vi "NI-SWITCH SwitchBlock Configuration.vi"(8 "error in (no error)":errorcluster, 11 "Reference In":refnum<k15>) -> (0 "error out":errorcluster, 1 "Analog Bus Array":string[](array[string]), 2 "Row Array":string[](array[string]), 3 "Reference out":refnum<k15>)   [LabVIEW 2019]
doc: "I. Description:\n\nThis is a subVI designed for use with NI SwitchBlock with NI-SWITCH. The purpose of this VI is to take in the NI SwitchBlock device, determine the number of rows and cards on the device, and generate a list of names for the rows and the analog bus lines on the NI SwitchBlock device\n\nII. Instructions for Running:\n\n1. Put your NI SWITCH reference into the control.\n2. Run the VI to produce two arrays of naming data for your NI SwitchBlock rows and analog buses.\n\nRefer to the NI Switches Help for the valid channel names and valid resource names for your switch module.\n\nIII. Block Diagram Steps:\n\n1.) Determine the model name, number of columns, and the number of rows from your NI SwitchBlock device.\n2.) Determine the number of cards on the NI SwitchBlock device by dividing the total number of columns, by the number of columns on each NI SwitchBlock card.\n3.) Use SwitchBlock Arrays.vi to find the names of the rows and analog buses on you device.\n\nIV. I/O Connections Overview:\n\nRefer to the NI Switches Getting Started Guide and NI Switches Help for information about connecting signals to your switch module."
uses:
  <resource>/objmgr/daqmx.rc
panel:
  out "Topology":string
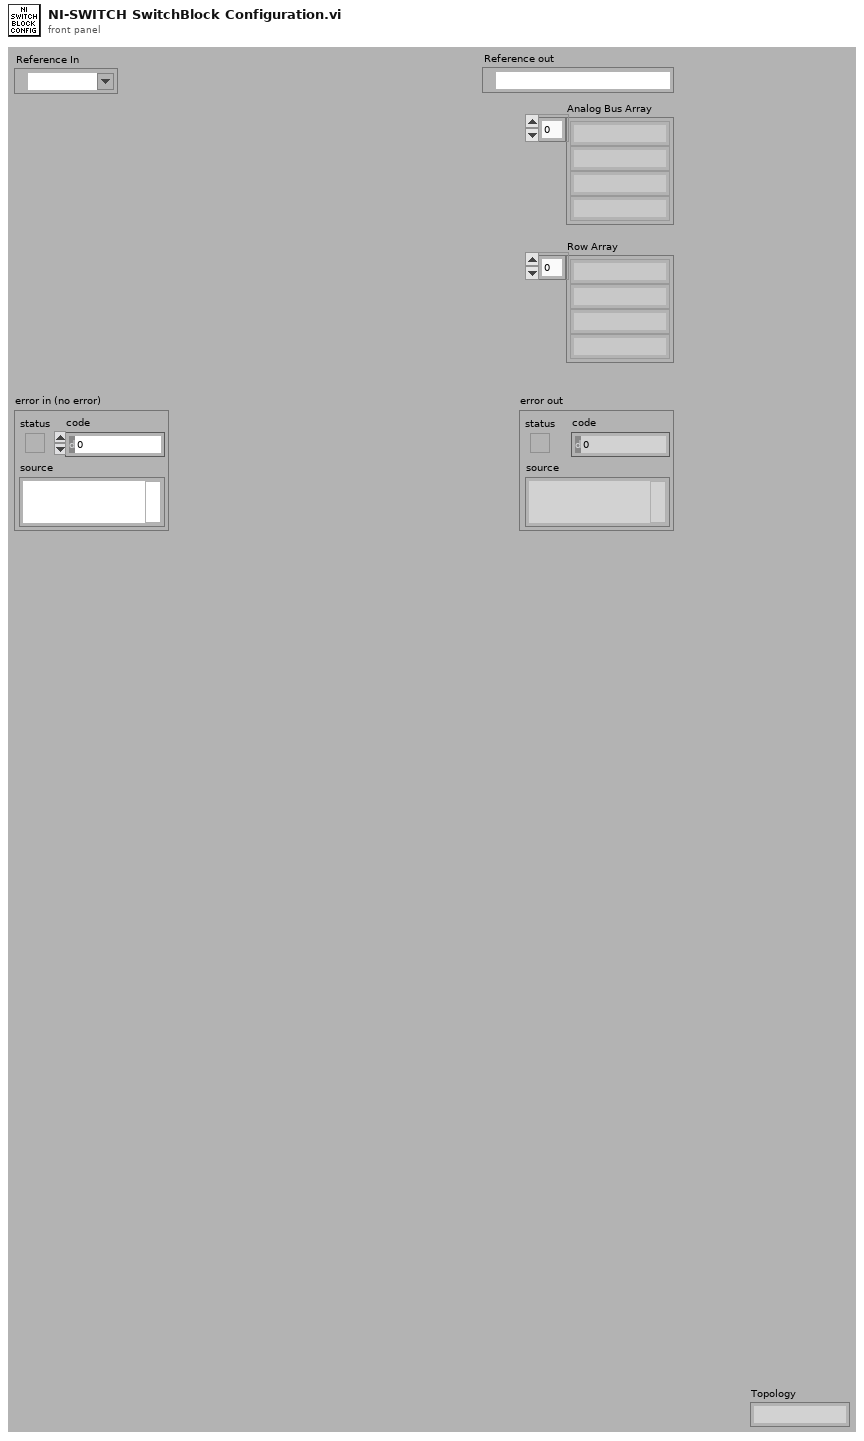
[diagram p1: front panel]
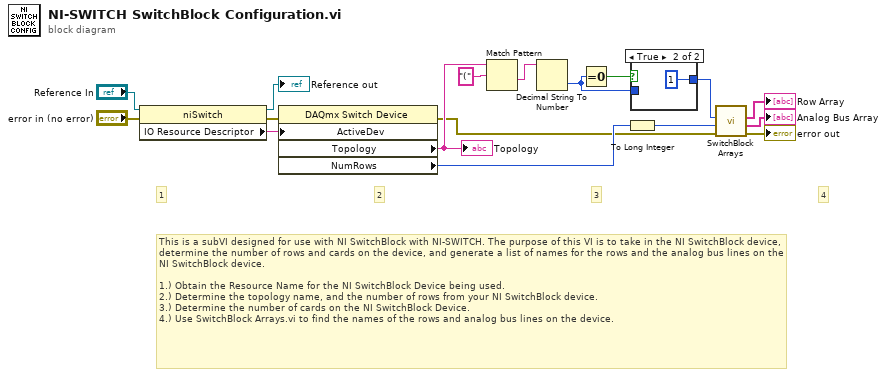
[diagram p0: block diagram]
diagram:
  # "4"
  # "3"
  # "2"
  # "1"
  # "This is a subVI designed for use with NI SwitchBlock with NI-SWITCH. The purpose of this VI is to take in the NI SwitchBlock device, determine the number of rows and cards on the device, and generate a list of names for the rows and the analog bus lines on the NI SwitchBlock device.\n\n1.) Obtain the Resource Name for the NI SwitchBlock Device being used.\n2.) Determine the topology name, and the number of rows from your NI SwitchBlock device.\n3.) Determine the number of cards on the NI SwitchBlock Device.\n4.) Use SwitchBlock Arrays.vi to find the names of the rows and analog bus lines on the device."
  n1 = property class="niSwitch"(reference="Reference In", error in="error in (no error)") -> (reference out=→"Reference out":refnum<k15>, error out=w4:errorcluster, "IO Resource Descriptor"=w5:string)
  n2 = property class="DAQmx Switch Device"(error in=w4, "ActiveDev"=w5) -> (error out=w1:errorcluster, "Topology"=w7:string, "NumRows"=w6:u32)  [unwired: 1 in, 1 out]
  "Topology" <- w7
  n3 = Match Pattern(string=w7, regular expression="(" ("string")) -> (after substring=w10:string)  [unwired: 1 in, 3 out]
  n4 = Decimal String To Number(string=w10) -> (number=w8:i32)  [unwired: 2 in, 1 out]
  n5 = Equal To 0?(x=w8) -> (x = 0?=w9:bool)
  n6 = To Long Integer(number=w6) -> (32bit integer=w2:i32)
  n7 = case shown="True" w9 {
    tunnel: [w18 1] -> w3
    tunnel: w8 -> [w18 _]
    frame False {
    }
    frame True {
    }
  }
  n8 = call "SwitchBlock Arrays.vi"("error in (no error)"=w1, "Number of Rows"=w2, "Number of Cards"=w3) -> ("error out"=→"error out":errorcluster, "Analog Bus Array"=→"Analog Bus Array":string[], "Row Array"=→"Row Array":string[])  [unwired: 6 in]
